vi "Table Logging Setting.vi"(4 "sample interval (ms)":i32=50, 6 "Log Length":i32=5, 7 "Log File path":path, 8 "error in (no error)":errorcluster, 9 "Logging Rate":T1=enum."30Hz", 10 "Data In":T2={"CommConnected_1"=FALSE, "Run_1?"=FALSE, "Fault_1?"=FALSE, "CommConnected_2"=FALSE, "Run_2?"=FALSE, "Fault_2?"=FALSE, "Motor Speed 2"=0.0, "Motor Speed_1"=28.0, "Motor Current_1"=0.0, "Motor Current_2"=0.0, "Motor1ConfigData"={"电机配置"=enum."配置1", "电压（V）"=0.0, "电流（A）"=0.0, "速度（RPM）"=0.0, "励磁方式"=enum."永磁"}, "Motor2ConfigData"={"电机配置"=enum."配置1", "电压（V）"=0.0, "电流（A）"=0.0, "速度（RPM）"=0.0, "励磁方式"=enum."永磁"}, "EmoStop_1?"=FALSE}, 11 "Record":bool) -> (0 "error out":errorcluster, 3 "Speed Log to Display":string[][](table)=[["2018-04-13 14:46:04", "8.0", "0.0", "0.0", "0.0"], ["2018-04-13 14:46:05", "9.0", "0.0", "0.0", "0.0"], ["2018-04-13 14:46:06", "10.0", "0.0", "0.0", "0.0"], ["2018-04-13 14:46:07", "11.0", "0.0", "0.0", "0.0"], ["2018-04-13 14:46:08", "12.0", "0.0", "0.0", "0.0"], ["2018-04-13 14:46:09", "13.0", "0.0", "0.0", "0.0"], ["2018-04-13 14:46:10", "14.0", "0.0", "0.0", "0.0"], ["2018-04-13 14:46:11", "15.0", "0.0", "0.0", "0.0"], ["2018-04-13 14:46:13", "17.0", "0.0", "0.0", "0.0"], ["2018-04-13 14:46:15", "19.0", "0.0", "0.0", "0.0"], ["2018-04-13 14:46:17", "21.0", "0.0", "0.0", "0.0"], ["2018-04-13 14:46:48", "3.0", "0.0", "0.0", "0.0"], ["2018-04-13 14:46:50", "5.0", "0.0", "0.0", "0.0"], ["2018-04-13 14:46:52", "7.0", "0.0", "0.0", "0.0"], ["2018-04-13 14:46:54", "9.0", "0.0", "0.0", "0.0"], ["2018-04-13 14:46:58", "13.0", "0.0", "0.0", "0.0"], ["2018-04-13 14:47:02", "17.0", "0.0", "0.0", "0.0"], ["2018-04-13 14:47:06", "21.0", "0.0", "0.0", "0.0"], ["2018-04-13 14:47:10", "25.0", "0.0", "0.0", "0.0"]])   [LabVIEW 2018]
uses:
  Ctls/DisplayIndicator.ctl
  Ctls/MotroConfigData.ctl
  Ctls/MotorConfig.ctl
  Ctls/MagType.ctl
  Ctls/LoggingRate.ctl
  Ctls/DatabaseCmd.ctl
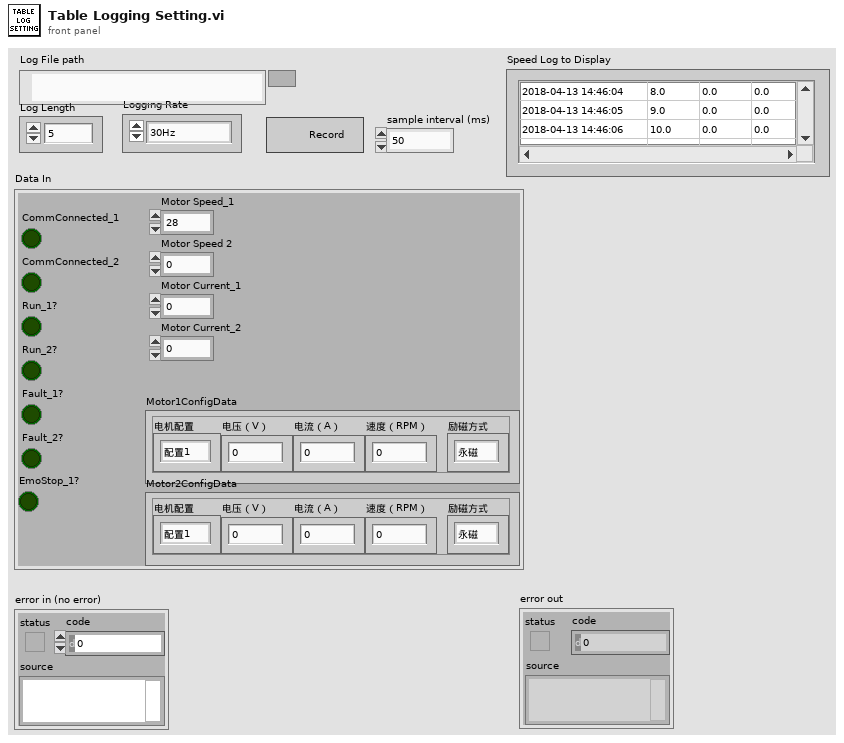
[diagram p1: front panel]
types:
  T1 = typedef "LoggingRate.ctl" = enum16{"1Hz", "5Hz", "10Hz", "20Hz", "30Hz", "40Hz"}
  T2 = typedef "DisplayIndicator.ctl" = cluster{"CommConnected_1":bool, "Run_1?":bool, "Fault_1?":bool, "CommConnected_2":bool, "Run_2?":bool, "Fault_2?":bool, "Motor Speed 2":sgl, "Motor Speed_1":sgl, "Motor Current_1":sgl, "Motor Current_2":sgl, "Motor1ConfigData":T3, "Motor2ConfigData":T3, "EmoStop_1?":bool}
  T3 = typedef "MotroConfigData.ctl" = cluster{"电机配置":T4, "电压（V）":dbl, "电流（A）":dbl, "速度（RPM）":dbl, "励磁方式":T5}
  T4 = typedef "MotorConfig.ctl" = enum16{"配置1", "配置2", "配置3", "配置4"}
  T5 = typedef "MagType.ctl" = enum16{"永磁", "励磁"}
  T6 = typedef "DatabaseCmd.ctl" = enum16{"Insert Table Title", "Add One Record", "Delete Record", "Get Table Records", "Clear"}
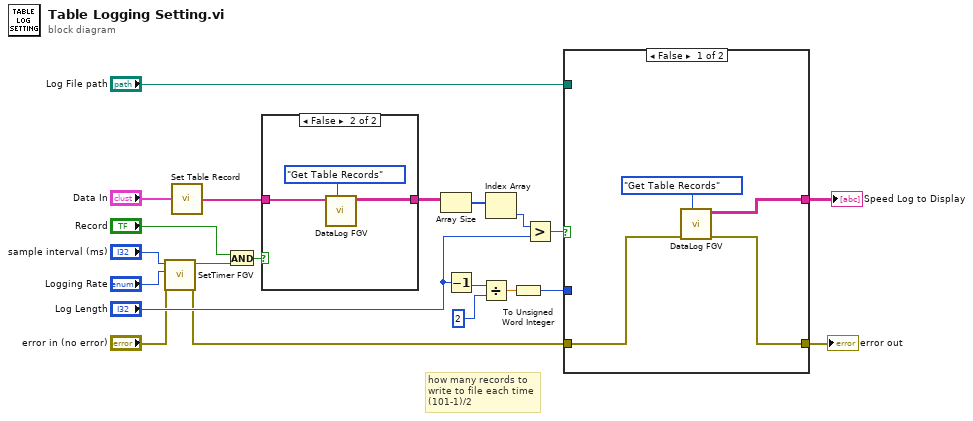
[diagram p0: block diagram]
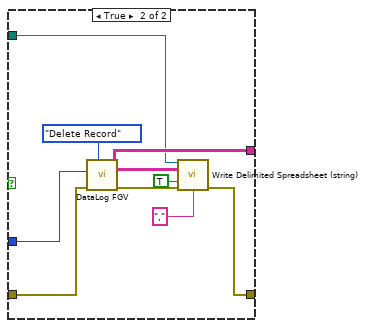
[diagram p2: hidden frame]
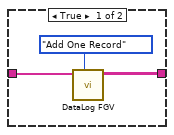
[diagram p3: hidden frame]
diagram:
  # "how many records to\nwrite to file each time\n(101-1)/2"
  n1 = call "SetTimer FGV.vi"("error in (no error)"="error in (no error)", "Logging Rate"="Logging Rate", "sample interval (ms)"="sample interval (ms)") -> ("error out"=w3:errorcluster, "Add?"=w18:bool)  [unwired: 7 in]
  n2 = call "Set Table Record.vi"("Data In"="Data In") -> ("Record Out"=w20:string[])
  n3 = And(x="Record", y=w18) -> (x .and. y?=w17:bool)
  n4 = case shown="False" w17 {
    tunnel: w20 -> [w24 w27]
    tunnel: [w23 w26] -> w5
    frame True {
      n5 = call "DataLog FGV.vi"("Method"=DatabaseCmd."Add One Record", "New Record"=w24) -> ("Speed Log"=w23:string[][])  [unwired: 7 in, 2 out]
    }
    frame False {
      n6 = call "DataLog FGV.vi"("Method"=DatabaseCmd."Get Table Records", "New Record"=w27) -> ("Speed Log"=w26:string[][])  [unwired: 7 in, 2 out]
    }
  }
  n7 = Array Size(array=w5) -> (size(s)=w16:i32[])
  n8 = Decrement(x="Log Length") -> (x-1=w12:i32)
  n9 = Divide(x=w12, y=2) -> (x/y=w10:dbl)
  n10 = Index Array(array=w16) -> (element=w15:i32)  [unwired: 1 in]
  n11 = To Unsigned Word Integer(number=w10) -> (unsigned 16bit integer=w9:u16)
  n12 = Greater?(x=w15, y="Log Length") -> (0:w14:bool)
  n13 = case shown="False" w14 {
    tunnel: w9 -> [_ w41]
    tunnel: [w29 w39] -> w8
    tunnel: w3 -> [w31 w36]
    tunnel: "Log File path" -> [_ w34]
    tunnel: [w28 w33] -> w6
    frame False {
      n14 = call "DataLog FGV.vi"("Method"=DatabaseCmd."Get Table Records", "error in (no error)"=w31) -> ("error out"=w28:errorcluster, "Speed Log"=w29:string[][])  [unwired: 7 in, 1 out]
    }
    frame True {
      n15 = call "DataLog FGV.vi"("Method"=DatabaseCmd."Delete Record", "error in (no error)"=w36, "length"=w41) -> ("error out"=w37:errorcluster, "log to file"=w38:string[][], "Speed Log"=w39:string[][])  [unwired: 6 in]
      n16 = call "Write Delimited Spreadsheet (string).vi"("Path"=w34, "2D data"=w38, "append to file?"=TRUE ("append to file? (new file:F)"), "error in"=w37, "delimiter (\\t)"="," ("delimiter (\\t)")) -> ("error out"=w33:errorcluster)  [unwired: 9 in, 1 out]
    }
  }
  "Speed Log to Display" <- w8
  "error out" <- w6
